vi "rawpower2totalprad.vi"(1 "PowerArray [W]":sgl[][](array[numeric]), 2 "No. of Samples\n[TOA / Sample Rate]":u32=10000, 3 "kbolott_and_volume":dbl[][](array[numeric])) -> (0 "final P_rad [MW]":dbl[](array[numeric]))   [LabVIEW 2014]
panel:
  in  "Nchannels":i32=32
  out "sample array [MW]":dbl[](array[numeric])
  out "constant":dbl
  out "full P_rad [MW]":dbl[](array[numeric])
  out "V_Cam":dbl format="%#_13g"
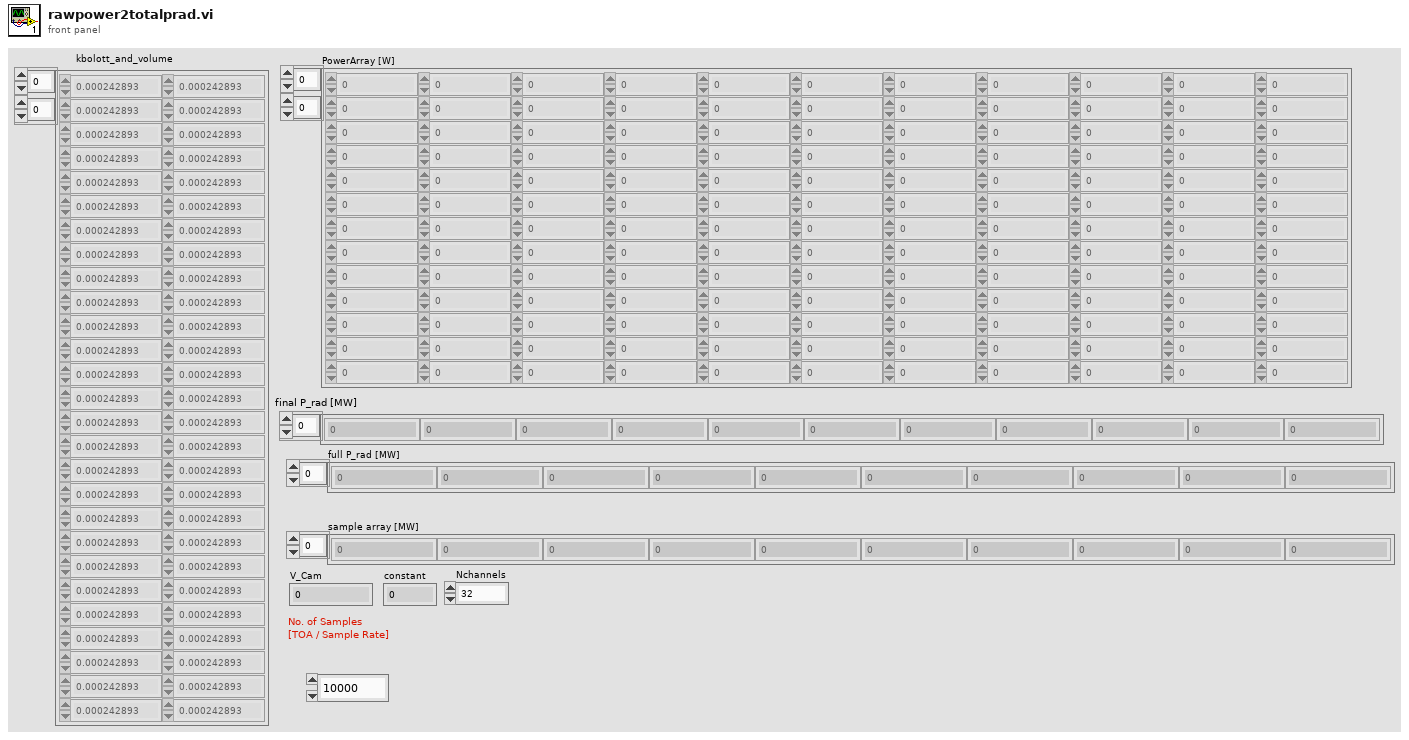
[diagram p1: front panel]
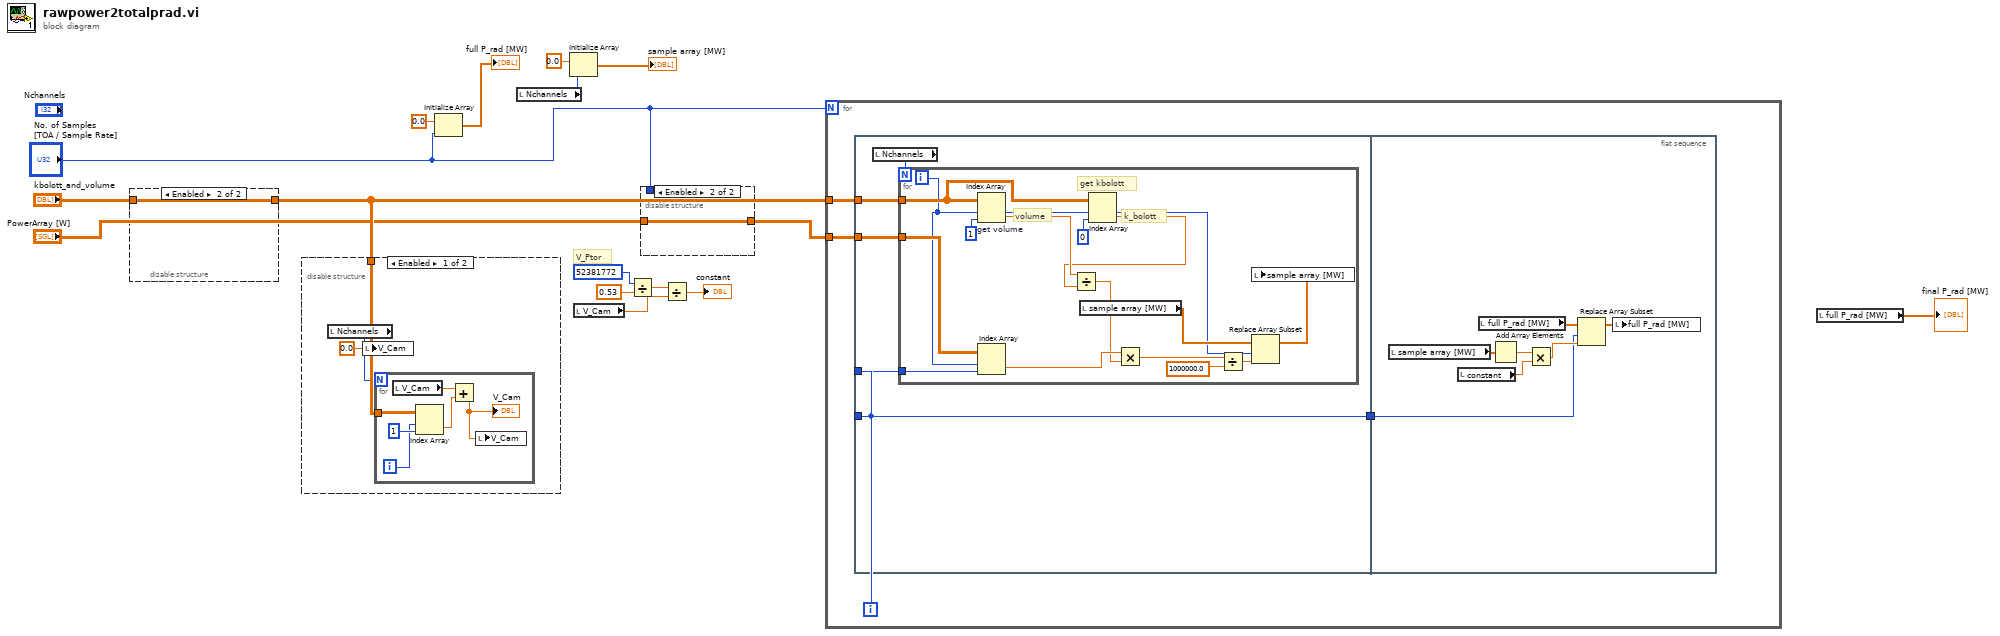
[diagram p0: block diagram]
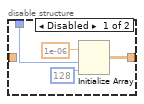
[diagram p2: hidden frame]
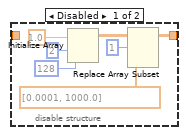
[diagram p3: hidden frame]
diagram:
  # "V_Ptor"
  n1 = disable-structure shown="Enabled" {
    disable-tunnel: [w17 w24] -> w3
    disable-tunnel: "kbolott_and_volume" -> [_ w24]
    frame Disabled {
      n2 = Initialize Array(1.0 ("element"), 2 ("dimension size"), 128 ("dimension size")) -> (w20:dbl[][])
      n3 = Replace Array Subset(array=w20, new element=dbl[] [0.0001, 1000.0] ("new element/subarray"), index (row)=1) -> (w17:dbl[][])  [unwired: 1 in]
    }
    frame Enabled {
    }
  }
  n4 = disable-structure shown="Enabled" {
    disable-tunnel: w3 -> [w27 _]
    frame Enabled {
      n5 = local read "Nchannels"() -> (w26:i32)
      n6 = local write "V_Cam"(0.0 ("V_Cam")) -> ()
      n7 = for {
        N: w26 -> [_]
        tunnel: w27 -> [w33]
        i -> [w29]
        n8 = local read "V_Cam"() -> (w32:dbl)
        n9 = Index Array(array=w33, index (row)=w29, index (col)=1 ("disabled index (col)")) -> (element=w31:dbl)
        n10 = Add(x=w32, y=w31) -> (x+y=w28:dbl)
        "V_Cam" <- w28
        n11 = local write "V_Cam"(w28) -> ()
      }
    }
    frame Disabled {
    }
  }
  n12 = Initialize Array(0.0 ("element"), "No. of Samples\n[TOA / Sample Rate]") -> (→"full P_rad [MW]":dbl[])
  n13 = local read "Nchannels"() -> (w12:i32)
  n14 = Initialize Array(0.0 ("element"), w12) -> (→"sample array [MW]":dbl[])
  n15 = local read "V_Cam"() -> (w7:dbl)
  n16 = Divide(x=52381772, y=0.53) -> (x/y=w8:dbl)
  n17 = disable-structure shown="Enabled" {
    disable-tunnel: "No. of Samples\n[TOA / Sample Rate]" -> [w36 _]
    disable-tunnel: [w34 w38] -> w4
    disable-tunnel: "PowerArray [W]" -> [_ w38]
    frame Disabled {
      n18 = Initialize Array(1e-06 ("element"), w36, 128 ("dimension size")) -> (w34:dbl[][])
    }
    frame Enabled {
    }
  }
  n19 = Divide(x=w8, y=w7) -> (x/y=→"constant":dbl)
  n20 = for {
    N: "No. of Samples\n[TOA / Sample Rate]" -> [_]
    tunnel: w4 -> [w42]
    tunnel: w3 -> [w41]
    i -> [w39]
    n21 = flat-sequence {
      tunnel: w42 -> [w46]
      tunnel: w41 -> [w45]
      tunnel: w39 -> [w44]
      tunnel: [w43] -> w40
      tunnel: w39 -> [w43]
      tunnel: w40 -> [w63]
      frame #0 {
        n22 = local read "Nchannels"() -> (w47:i32)
        n23 = for {
          N: w47 -> [_]
          tunnel: w46 -> [w59]
          tunnel: w45 -> [w61]
          tunnel: w44 -> [w55]
          i -> [w57]
          # "get kbolott"
          # "k_bolott"
          # "volume"
          n24 = Index Array "get volume"(array=w61, index (row)=w57, index (col)=1 ("disabled index (col)")) -> (element=w52:dbl)
          n25 = Index Array(array=w59, index (row)=w57, index (col)=w55) -> (element=w50:sgl)
          n26 = local read "sample array [MW]"() -> (w58:dbl[])
          n27 = Index Array(array=w61, index (row)=w57, index (col)=0 ("disabled index (col)")) -> (element=w51:dbl)
          n28 = Divide(x=w52, y=w51) -> (x/y=w49:dbl)
          n29 = Multiply(x=w50, y=w49) -> (x*y=w48:dbl)
          n30 = Divide(x=w48, y=1000000.0) -> (x/y=w53:dbl)
          n31 = Replace Array Subset(array=w58, new element=w53, index=w57) -> (w56:dbl[])
          n32 = local write "sample array [MW]"(w56) -> ()
        }
      }
      frame #1 {
        n33 = local read "sample array [MW]"() -> (w64:dbl[])
        n34 = local read "constant"() -> (w66:dbl)
        n35 = local read "full P_rad [MW]"() -> (w67:dbl[])
        n36 = Add Array Elements(numeric array=w64) -> (sum=w65:dbl)
        n37 = Multiply(x=w65, y=w66) -> (x*y=w68:dbl)
        n38 = Replace Array Subset(array=w67, new element=w68, index=w63) -> (w69:dbl[])
        n39 = local write "full P_rad [MW]"(w69) -> ()
      }
    }
  }
  n40 = local read "full P_rad [MW]"() -> (→"final P_rad [MW]":dbl[])
